vi "compileDigitalOutputList.vi"(8 "error in (no error)":errorcluster, 11 "ScriptListCompiler in":refnum<class "ScriptListCompiler.lvclass">) -> (0 "error out":errorcluster, 3 "ScriptListCompiler out":refnum<class "ScriptListCompiler.lvclass">)   [LabVIEW 2011, in "Compiler.lvlib" / "ScriptListCompiler.lvclass"]
doc: "Compiles the Digital ScriptList.\n i) Adds the additional digital events to the Digital ScriptList.\n ii) Splits Digital List into devices.\n iii) Produces digital trigger pulses for each digital device, and add them to\n the relavent ScriptList.\n iv) Apply digital delays.\n v) Apply pulse finishing and calibrate all digital data.\n vi) Adds new data to each device script list."
uses:
  ScriptListCompiler.lvclass
  ScriptListCompiler.lvclass/ScriptListCompiler.ctl
  DatabaseHelpers/Database Objects/device/device.lvclass
  DatabaseHelpers/Database Objects/DeviceArray/DeviceArray.lvclass
  Scripting/ScriptingEvent/ScriptEventList/ScriptEventList.lvclass
  DatabaseHelpers/DbConnection/DeviceDataBase/deviceDataBase.lvclass
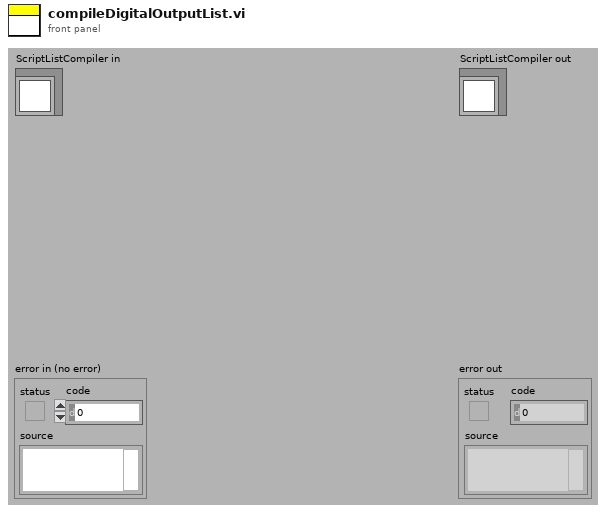
[diagram p1: front panel]
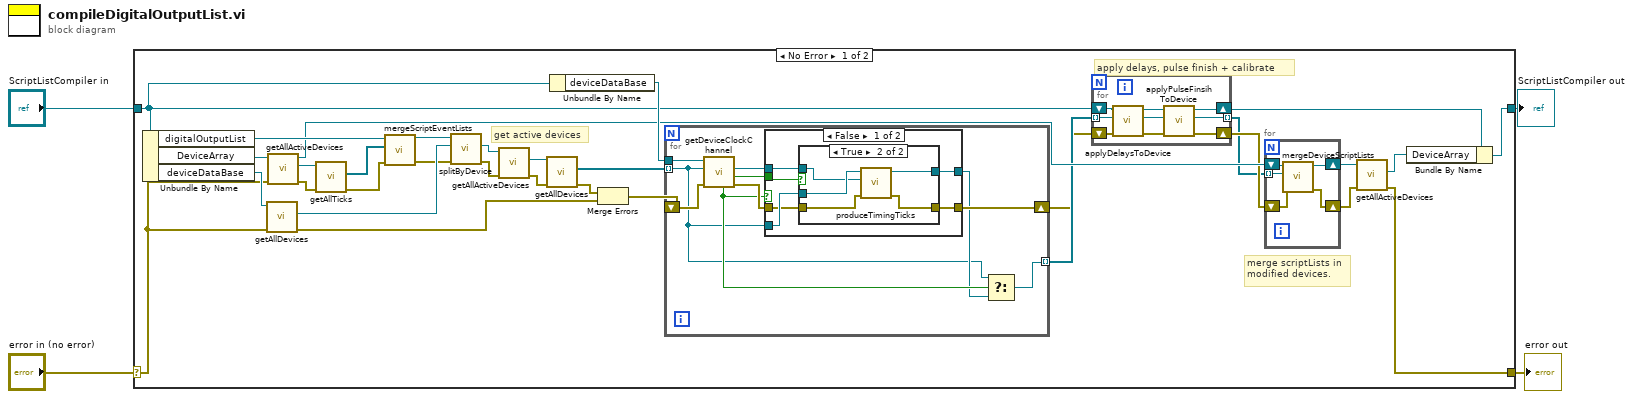
[diagram p0: block diagram]
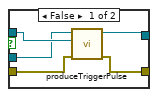
[diagram p2: hidden frame]
diagram:
  n1 = case shown="No Error" "error in (no error)" {
    selector: "error in (no error)" -> [w27 w79]
    tunnel: [w6 w79] -> w3
    tunnel: [w16 w78] -> w1
    tunnel: "ScriptListCompiler in" -> [w14 w78]
    frame No Error {
      # "apply delays, pulse finish + calibrate"
      # "get active devices"
      # "merge scriptLists in\nmodified devices."
      n2 = Unbundle By Name(w14) -> ("digitalOutputList"=w32:refnum<class "ScriptEventList.lvclass">, "DeviceArray"=w36:refnum<class "DeviceArray.lvclass">, "deviceDataBase"=w28:refnum<class "deviceDataBase.lvclass">)
      n3 = call "getAllDevices.vi"("error in (no error)"=w27, "deviceDataBase in"=w28) -> ("error out"=w19:errorcluster, "deviceArray.lvclass"=w29:refnum<class "DeviceArray.lvclass">)  [unwired: 7 in, 1 out]
      n4 = call "getAllActiveDevices.vi"("error in (no error)"=w27, "DeviceArray in"=w36) -> ("error out"=w34:errorcluster, "DeviceArray"=w35:refnum<class "DeviceArray.lvclass">, "DeviceArray out"=w15:refnum<class "DeviceArray.lvclass">)  [unwired: 7 in]
      n5 = call "getAllTicks.vi"("error in (no error)"=w34, "DeviceArray in"=w35) -> ("error out"=w31:errorcluster, "scriptEventListArray"=w33:refnum<class "ScriptEventList.lvclass">[])  [unwired: 7 in, 1 out]
      n6 = call "mergeScriptEventLists.vi"("error in (no error)"=w31, "Array"=w33, "ScriptEventList in"=w32) -> ("error out"=w26:errorcluster, "ScriptEventList out"=w30:refnum<class "ScriptEventList.lvclass">)  [unwired: 7 in]
      n7 = call "splitByDevice.vi"("error in (no error)"=w26, "DeviceArray"=w29, "ScriptEventList in"=w30) -> ("error out"=w17:errorcluster, "DeviceArray out"=w18:refnum<class "DeviceArray.lvclass">)  [unwired: 6 in, 1 out]
      n8 = call "getAllActiveDevices.vi"("error in (no error)"=w17, "DeviceArray in"=w18) -> ("error out"=w24:errorcluster, "DeviceArray"=w25:refnum<class "DeviceArray.lvclass">)  [unwired: 7 in, 1 out]
      n9 = call "getAllDevices.vi"("error in (no error)"=w24, "DeviceArray.lvclass in"=w25) -> ("error out"=w23:errorcluster, "deviceArray"=w21:refnum<class "device.lvclass">[])  [unwired: 7 in, 1 out]
      n10 = Unbundle By Name(w14) -> ("deviceDataBase"=w20:refnum<class "deviceDataBase.lvclass">)
      n11 = Merge Errors(w23, w19) -> (w22:errorcluster)
      n12 = for {
        tunnel: w21 -> [w52] mode=indexing
        shift-right: [w55] -> w11
        shift-left: w22 -> [w60]
        tunnel: w20 -> [w59]
        tunnel: [w51] -> w12 mode=indexing
        n13 = call "getDeviceClockChannel.vi"("error in (no error)"=w60, "device"=w52, "deviceDataBase in"=w59) -> ("error out"=w56:errorcluster, "isClock"=w58:bool, "timingChannel"=w57:refnum<class "Channel.lvclass">, "noChannel"=w54:bool)  [unwired: 4 in, 1 out]
        n14 = case shown="False" w54 {
          tunnel: w58 -> [w66 _]
          tunnel: w57 -> [w65 _]
          tunnel: w52 -> [w64 _]
          tunnel: w56 -> [w63 w77]
          tunnel: [w62 w77] -> w55
          tunnel: [w61 _] -> w53
          frame False {
            n15 = case shown="True" w66 {
              tunnel: w65 -> [w70 w75]
              tunnel: w64 -> [w69 w76]
              tunnel: w63 -> [w68 w74]
              tunnel: [w67 w73] -> w62
              tunnel: [w71 w72] -> w61
              frame False {
                n16 = call "produceTriggerPulse.vi"("error in (no error)"=w68, "Channel"=w70, "device in"=w69) -> ("error out"=w67:errorcluster, "device out"=w71:refnum<class "device.lvclass">)  [unwired: 7 in]
              }
              frame True {
                n17 = call "produceTimingTicks.vi"("error in (no error)"=w74, "Channel"=w75, "device in"=w76) -> ("error out"=w73:errorcluster, "device out"=w72:refnum<class "device.lvclass">)  [unwired: 7 in]
              }
            }
          }
          frame True {
          }
        }
        n18 = Select(t=w52, s=w54, f=w53) -> (s? t:f=w51:refnum<class "device.lvclass">)
      }
      n19 = for {
        tunnel: w12 -> [w44] mode=indexing
        shift-right: [w41] -> w13
        shift-left: w14 -> [w45]
        shift-right: [w37] -> w10
        shift-left: w11 -> [w43]
        tunnel: [w40] -> w9 mode=indexing
        n20 = call "applyDelaysToDevice.vi"("error in (no error)"=w43, "device"=w44, "ScriptListCompiler in"=w45) -> ("error out"=w38:errorcluster, "device out"=w39:refnum<class "device.lvclass">, "ScriptListCompiler out"=w42:refnum<class "ScriptListCompiler.lvclass">)  [unwired: 6 in]
        n21 = call "applyPulseFinsihToDevice.vi"("error in (no error)"=w38, "device"=w39, "ScriptListCompiler in"=w42) -> ("error out"=w37:errorcluster, "device out"=w40:refnum<class "device.lvclass">, "ScriptListCompiler out"=w41:refnum<class "ScriptListCompiler.lvclass">)  [unwired: 6 in]
      }
      n22 = for {
        shift-right: [w49] -> w8
        shift-left: w15 -> [w50]
        tunnel: w9 -> [w46] mode=indexing
        shift-right: [w47] -> w7
        shift-left: w10 -> [w48]
        n23 = call "mergeDeviceScriptLists.vi"("error in (no error)"=w48, "device"=w46, "DeviceArray in"=w50) -> ("error out"=w47:errorcluster, "DeviceArray out"=w49:refnum<class "DeviceArray.lvclass">)  [unwired: 7 in]
      }
      n24 = call "getAllActiveDevices.vi"("error in (no error)"=w7, "DeviceArray in"=w8) -> ("error out"=w6:errorcluster, "DeviceArray"=w5:refnum<class "DeviceArray.lvclass">)  [unwired: 7 in, 1 out]
      n25 = Bundle By Name(cluster=w13, "DeviceArray"=w5) -> (w16:refnum<class "ScriptListCompiler.lvclass">)
    }
    frame Error {
    }
  }
  "error out" <- w3
  "ScriptListCompiler out" <- w1
